vi "Read Signal Amplitude from State.vi"(8 "error in (no error)":errorcluster, 11 "SV Signal in":refnum<class "SV Signal.lvclass">) -> (0 "error out":errorcluster, 2 "amplitude":dbl, 3 "SV Signal out":refnum<class "SV Signal.lvclass">)   [LabVIEW 2017, in "SV Signal.lvclass"]
uses:
  <vilib>/addons/_NISVFA/_Generation/Signal Generation/SV Signal/SV Signal.lvclass
  <vilib>/addons/_NISVFA/_Generation/Signal Generation/SV Signal/SV Signal.lvclass/SV Signal.ctl
  <vilib>/addons/_NISVFA/_Generation/Signal Generation/SV Signal/sv_Signal State Attribute.ctl
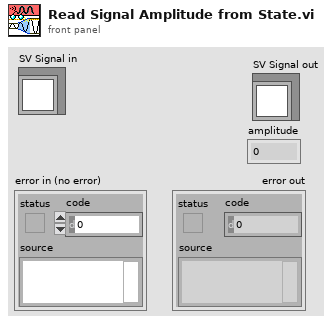
[diagram p1: front panel]
types:
  T1 = typedef "SV Signal.lvclass/sv_Signal State Attribute.ctl" = string
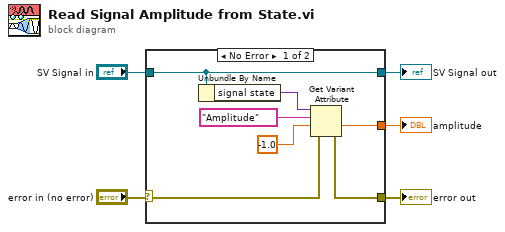
[diagram p0: block diagram]
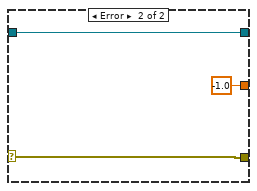
[diagram p2: hidden frame]
diagram:
  n1 = case shown="No Error" "error in (no error)" {
    selector: "error in (no error)" -> [w7 w15]
    tunnel: [w10 w15] -> w5
    tunnel: [w8 -1.0 ("amplitude")] -> w4
    tunnel: "SV Signal in" -> [w6 w14]
    tunnel: [w6 w14] -> w1
    frame No Error {
      n2 = Unbundle By Name(w6) -> ("signal state"=w11:variant)
      n3 = Get Variant Attribute(Variant=w11, name=T1 "Amplitude", default value (empty Variant)=-1.0 ("amplitude"), error in=w7) -> (value=w8:dbl, error out=w10:errorcluster)  [unwired: 2 out]
    }
    frame Error {
    }
  }
  "amplitude" <- w4
  "SV Signal out" <- w1
  "error out" <- w5
